vi "Generate_WayPoints_STOPMEASURE.vi"(8 "Update Position Loop Wait Time (us)":u32=50000, 11 "Input Cluster":T2={"Scan Rate (um/s)"=15.0, "X Start"=15.0, "X End"=15.0, "Y Start"=15.0, "Y End"=15.0, " Z Start"=15.0, "Number of Lines"=15, "V"=15.0, "Z End"=15.0, "Approach Rate (um/s)"=15.0, "Squish Approach Rate (um/s)"=15.0, "V 2"=15.0, "StopMeasureDist (um)"=15.0, "HoldTimer / us"=0}) -> (0 "output cluster":T1)   [LabVIEW 2023]
uses:
  TypeDefs/WayPointCluster.ctl
panel:
  in  "WayPointCluster":T1
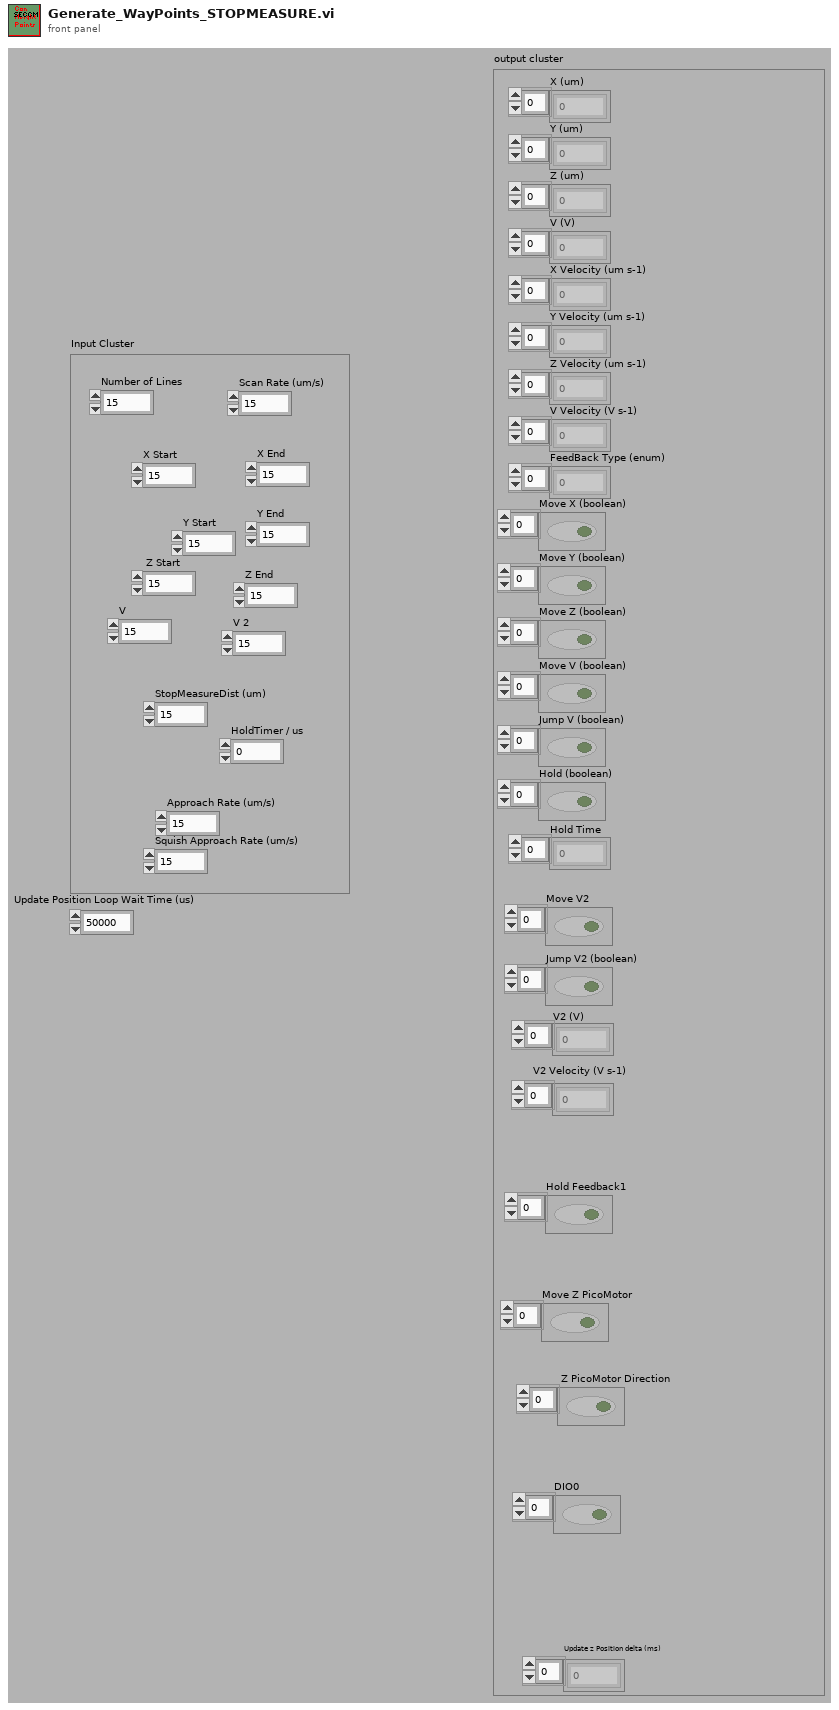
[diagram p1: front panel]
types:
  T1 = typedef "WayPointCluster.ctl" = cluster{"X (um)":dbl[], "Y (um)":dbl[], "Z (um)":dbl[], "V (V)":dbl[], "X Velocity (um s-1)":dbl[], "Y Velocity (um s-1)":dbl[], "Z Velocity (um s-1)":dbl[], "V Velocity (V s-1)":dbl[], "FeedBack Type (enum)":u16[], "Move X (boolean)":bool[], "Move Y (boolean)":bool[], "Move Z (boolean)":bool[], "Move V (boolean)":bool[], "Jump V (boolean)":bool[], "Hold (boolean)":bool[], "Hold Time":u32[], "V2 (V)":dbl[], "Move V2":bool[], "V2 Velocity (V s-1)":dbl[], "Jump V2 (boolean)":bool[], "Update z Position delta (ms)":i16[], "Hold Feedback1":bool[], "Move Z PicoMotor":bool[], " Z PicoMotor Direction":bool[], "DIO0":bool[]}
  T2 = cluster{"Scan Rate (um/s)":dbl, "X Start":dbl, "X End":dbl, "Y Start":dbl, "Y End":dbl, " Z Start":dbl, "Number of Lines":u32, "V":dbl, "Z End":dbl, "Approach Rate (um/s)":dbl, "Squish Approach Rate (um/s)":dbl, "V 2":dbl, "StopMeasureDist (um)":dbl, "HoldTimer / us":u32}
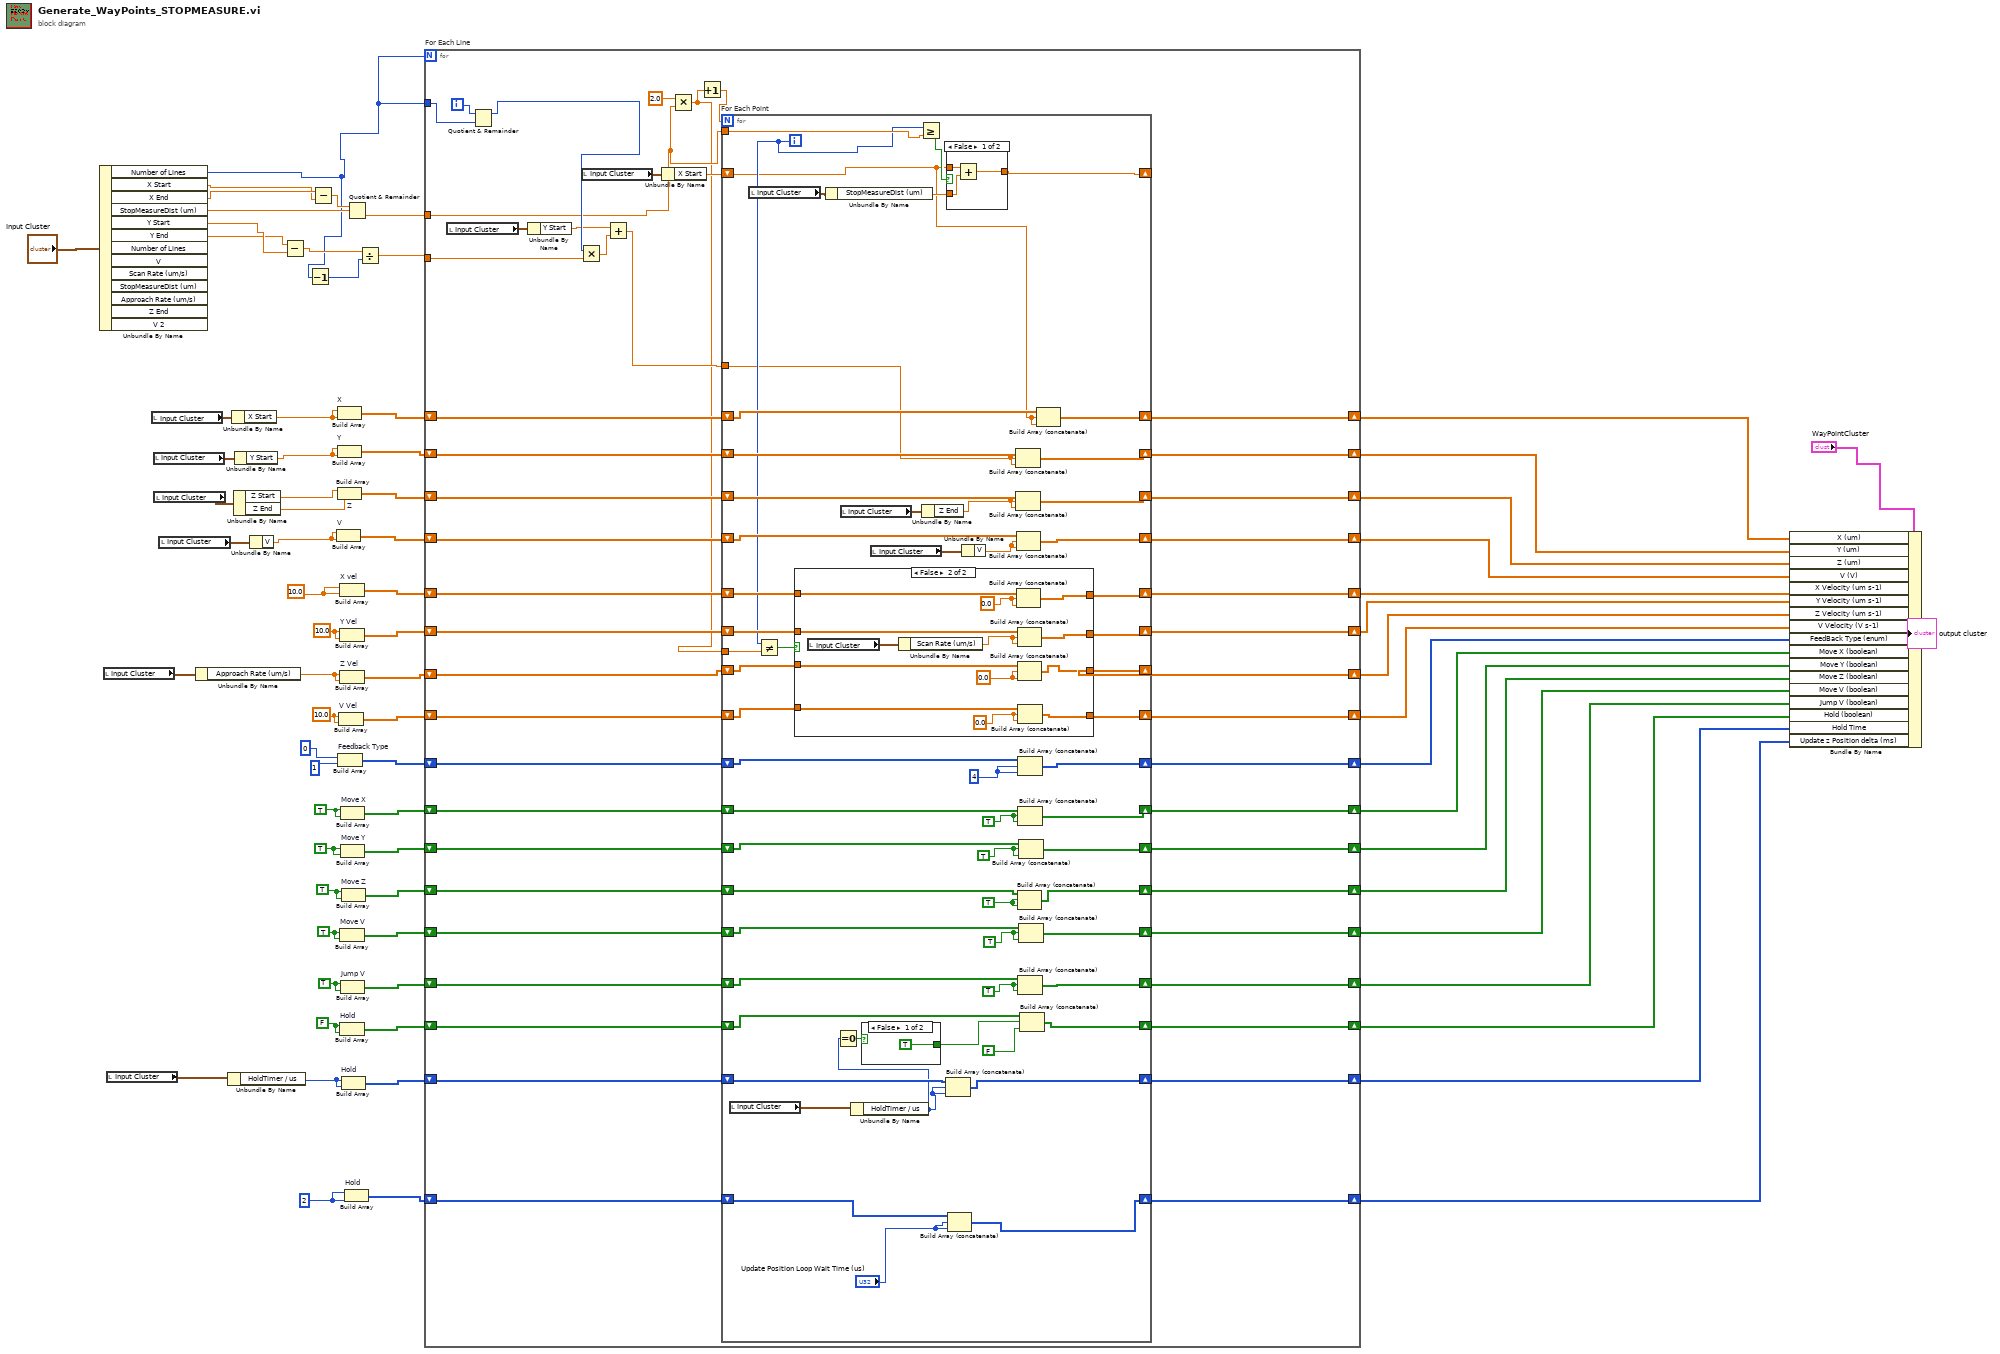
[diagram p0: block diagram]
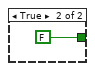
[diagram p2: hidden frame]
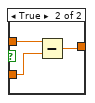
[diagram p3: hidden frame]
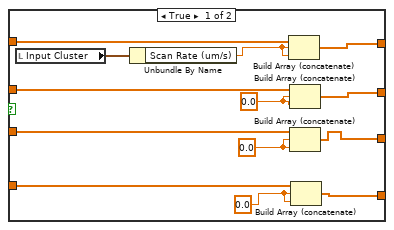
[diagram p4: hidden frame]
diagram:
  w3 = u32 2 ("element")
  w8 = FALSE
  w9 = TRUE
  w10 = TRUE
  w11 = TRUE
  w12 = TRUE
  w13 = TRUE
  w15 = 10.0 ("element")
  w17 = 10.0 ("element")
  w18 = 10.0 ("element")
  n1 = Unbundle By Name("Input Cluster") -> ("Number of Lines"=w64:u32, "X Start"=w62:dbl, "X End"=w72:dbl, "StopMeasureDist (um)"=w70:dbl, "Y Start"=w68:dbl, "Y End"=w67:dbl)  [unwired: 7 out]
  n2 = local read "Input Cluster"() -> (w41:T2)
  n3 = local read "Input Cluster"() -> (w35:T2)
  n4 = local read "Input Cluster"() -> (w45:T2)
  n5 = local read "Input Cluster"() -> (w44:T2)
  n6 = local read "Input Cluster"() -> (w43:T2)
  n7 = local read "Input Cluster"() -> (w42:T2)
  n8 = Unbundle By Name(w41) -> ("Approach Rate (um/s)"=w16:dbl)
  n9 = Unbundle By Name(w35) -> ("HoldTimer / us"=w7:u32)
  n10 = Unbundle By Name(w45) -> ("X Start"=w22:dbl)
  n11 = Unbundle By Name(w43) -> ("Z Start"=w20:dbl, "Z End"=w6:dbl)
  n12 = Unbundle By Name(w44) -> ("Y Start"=w21:dbl)
  n13 = Unbundle By Name(w42) -> ("V"=w19:dbl)
  n14 = Subtract(x=w67, y=w68) -> (x-y=w66:dbl)
  n15 = Decrement(x=w64) -> (x-1=w63:u32)
  n16 = Subtract(x=w72, y=w62) -> (x-y=w71:dbl)
  n17 = Build Array "V"(w19, w19) -> (w57:dbl[])
  n18 = Build Array "X"(w22, w22) -> (w60:dbl[])
  n19 = Build Array "Y"(w21, w21) -> (w59:dbl[])
  n20 = Build Array "Z"(w20, w6) -> (w58:dbl[])
  n21 = Build Array "Feedback Type"(u16 0 ("element"), u16 1 ("element")) -> (w52:u16[])
  n22 = Build Array "V Vel"(w15, w15) -> (w53:dbl[])
  n23 = Build Array "X vel"(w18, w18) -> (w56:dbl[])
  n24 = Build Array "Y Vel"(w17, w17) -> (w55:dbl[])
  n25 = Build Array "Z Vel"(w16, w16) -> (w54:dbl[])
  n26 = Build Array "Move V"(w10, w10) -> (w48:bool[])
  n27 = Build Array "Hold"(w8, w8) -> (w46:bool[])
  n28 = Build Array "Move X"(w13, w13) -> (w51:bool[])
  n29 = Build Array "Move Y"(w12, w12) -> (w50:bool[])
  n30 = Build Array "Jump V"(w9, w9) -> (w47:bool[])
  n31 = Build Array "Move Z"(w11, w11) -> (w49:bool[])
  n32 = Build Array "Hold"(w7, w7) -> (w36:u32[])
  n33 = Build Array "Hold"(w3, w3) -> (w2:u32[])
  n34 = Quotient & Remainder(x=w71, y=w70) -> (floor(x/y)=w69:dbl)  [unwired: 1 out]
  n35 = Divide(x=w66, y=w63) -> (x/y=w65:dbl)
  n36 = for "For Each Line" {
    N: w64 -> [_]
    tunnel: w69 -> [w79]
    tunnel: w64 -> [w120]
    tunnel: w65 -> [w119]
    shift-right: [w112] -> w40
    shift-left: w60 -> [w113]
    shift-right: [w97] -> w39
    shift-left: w59 -> [w111]
    shift-right: [w96] -> w38
    shift-left: w58 -> [w110]
    shift-right: [w95] -> w37
    shift-left: w57 -> [w109]
    shift-right: [w94] -> w34
    shift-left: w56 -> [w108]
    shift-right: [w93] -> w33
    shift-left: w55 -> [w107]
    shift-right: [w92] -> w32
    shift-left: w54 -> [w106]
    shift-right: [w91] -> w31
    shift-left: w53 -> [w105]
    shift-right: [w90] -> w30
    shift-left: w52 -> [w104]
    shift-right: [w89] -> w29
    shift-left: w51 -> [w103]
    shift-right: [w88] -> w28
    shift-left: w50 -> [w102]
    shift-right: [w87] -> w27
    shift-left: w49 -> [w101]
    shift-right: [w86] -> w26
    shift-left: w48 -> [w100]
    shift-right: [w85] -> w25
    shift-left: w47 -> [w99]
    shift-right: [w84] -> w24
    shift-left: w46 -> [w98]
    shift-right: [w76] -> w23
    shift-left: w36 -> [w77]
    shift-right: [w74] -> w1
    shift-left: w2 -> [w75]
    i -> [w121]
    n37 = local read "Input Cluster"() -> (w116:T2)
    n38 = Quotient & Remainder(x=w121, y=w120) -> (x-y*floor(x/y)=w118:u32)  [unwired: 1 out]
    n39 = Unbundle By Name(w116) -> ("Y Start"=w115:dbl)
    n40 = Multiply(x=w118, y=w119) -> (x*y=w117:dbl)
    n41 = local read "Input Cluster"() -> (w82:T2)
    n42 = Add(x=w115, y=w117) -> (x+y=w114:dbl)
    n43 = Unbundle By Name(w82) -> ("X Start"=w81:dbl)
    n44 = Multiply(x=2.0, y=w79) -> (x*y=w78:dbl)
    n45 = Increment(x=w78) -> (x+1=w80:dbl)
    n46 = for "For Each Point" {
      N: w80 -> [_]
      tunnel: w114 -> [w140]
      shift-right: [w179] -> w112
      shift-left: w113 -> [w180]
      shift-right: [w177] -> w97
      shift-left: w111 -> [w178]
      shift-right: [w175] -> w96
      shift-left: w110 -> [w176]
      shift-right: [w173] -> w95
      shift-left: w109 -> [w174]
      shift-right: [w171] -> w94
      shift-left: w108 -> [w172]
      shift-right: [w169] -> w93
      shift-left: w107 -> [w170]
      shift-right: [w167] -> w92
      shift-left: w106 -> [w168]
      shift-right: [w166] -> w91
      shift-left: w105 -> [w158]
      shift-right: [w165] -> w90
      shift-left: w104 -> [w157]
      shift-right: [w164] -> w89
      shift-left: w103 -> [w156]
      shift-right: [w163] -> w88
      shift-left: w102 -> [w155]
      shift-right: [w162] -> w87
      shift-left: w101 -> [w154]
      shift-right: [w161] -> w86
      shift-left: w100 -> [w153]
      shift-right: [w160] -> w85
      shift-left: w99 -> [w152]
      shift-right: [w159] -> w84
      shift-left: w98 -> [w151]
      tunnel: w78 -> [w147]
      shift-right: [w145] -> _
      shift-left: w81 -> [w141]
      tunnel: w79 -> [w144]
      shift-right: [w129] -> w76
      shift-left: w77 -> [w130]
      shift-right: [w125] -> w74
      shift-left: w75 -> [w127]
      i -> [w142]
      w132 = TRUE
      w133 = TRUE
      w134 = TRUE
      w135 = TRUE
      w136 = TRUE
      w137 = u16 4 ("element")
      n47 = local read "Input Cluster"() -> (w128:T2)
      n48 = local read "Input Cluster"() -> (w181:T2)
      n49 = Not Equal?(x=w142, y=w147) -> (x != y?=w148:bool)
      n50 = case shown="False" w148 {
        tunnel: w172 -> [w202 w215]
        tunnel: [w201 w214] -> w171
        tunnel: w170 -> [w200 w213]
        tunnel: [w199 w212] -> w169
        tunnel: w168 -> [w198 w211]
        tunnel: [w197 w210] -> w167
        tunnel: [w196 w209] -> w166
        tunnel: w158 -> [w195 w208]
        frame True {
          w190 = 0.0 ("element")
          w191 = 0.0 ("element")
          w192 = 0.0 ("element")
          n51 = local read "Input Cluster"() -> (w194:T2)
          n52 = Unbundle By Name(w194) -> ("Scan Rate (um/s)"=w193:dbl)
          n53 = Build Array (concatenate) ("X")(w202, w193, w193) -> (w201:dbl[])
          n54 = Build Array (concatenate) ("X")(w200, w192, w192) -> (w199:dbl[])
          n55 = Build Array (concatenate) ("X")(w198, w191, w191) -> (w197:dbl[])
          n56 = Build Array (concatenate) ("X")(w195, w190, w190) -> (w196:dbl[])
        }
        frame False {
          w203 = 0.0 ("element")
          w204 = 0.0 ("element")
          w206 = 0.0 ("element")
          n57 = local read "Input Cluster"() -> (w207:T2)
          n58 = Unbundle By Name(w207) -> ("Scan Rate (um/s)"=w205:dbl)
          n59 = Build Array (concatenate) ("X")(w215, w206, w206) -> (w214:dbl[])
          n60 = Build Array (concatenate) ("X")(w213, w205, w205) -> (w212:dbl[])
          n61 = Build Array (concatenate) ("X")(w211, w204, w204) -> (w210:dbl[])
          n62 = Build Array (concatenate) ("X")(w208, w203, w203) -> (w209:dbl[])
        }
      }
      n63 = Unbundle By Name(w181) -> ("StopMeasureDist (um)"=w146:dbl)
      n64 = local read "Input Cluster"() -> (w150:T2)
      n65 = Unbundle By Name(w128) -> ("HoldTimer / us"=w122:u32)
      n66 = Equal To 0?(x=w122) -> (x = 0?=w123:bool)
      n67 = case shown="False" w123 {
        tunnel: [TRUE FALSE] -> w124
        frame False {
        }
        frame True {
        }
      }
      n68 = local read "Input Cluster"() -> (w149:T2)
      n69 = Greater Or Equal?(x=w142, y=w144) -> (x >= y?=w143:bool)
      n70 = Unbundle By Name(w150) -> ("Z End"=w139:dbl)
      n71 = Build Array (concatenate) ("X")(w130, w122, w122) -> (w129:u32[])
      n72 = case shown="False" w143 {
        tunnel: w146 -> [w186 w189]
        tunnel: w141 -> [w185 w187]
        tunnel: [w184 w188] -> w145
        frame False {
          n73 = Add(x=w185, y=w186) -> (x+y=w184:dbl)
        }
        frame True {
          n74 = Subtract(x=w187, y=w189) -> (x-y=w188:dbl)
        }
      }
      n75 = Build Array (concatenate) ("X")(w127, "Update Position Loop Wait Time (us)", "Update Position Loop Wait Time (us)") -> (w125:u32[])
      n76 = Unbundle By Name(w149) -> ("V"=w138:dbl)
      n77 = Build Array (concatenate) ("X")(w178, w140, w140) -> (w177:dbl[])
      n78 = Build Array (concatenate) ("X")(w176, w139, w139) -> (w175:dbl[])
      n79 = Build Array (concatenate) ("X")(w174, w138, w138) -> (w173:dbl[])
      n80 = Build Array (concatenate) ("X")(w154, w134, w134) -> (w162:bool[])
      n81 = Build Array (concatenate) ("X")(w157, w137, w137) -> (w165:u16[])
      n82 = Build Array (concatenate) ("X")(w156, w136, w136) -> (w164:bool[])
      n83 = Build Array (concatenate) ("X")(w152, w132, w132) -> (w160:bool[])
      n84 = Build Array (concatenate) ("X")(w155, w135, w135) -> (w163:bool[])
      n85 = Build Array (concatenate) ("X")(w153, w133, w133) -> (w161:bool[])
      n86 = Build Array (concatenate) ("X")(w151, w124, FALSE) -> (w159:bool[])
      n87 = Build Array (concatenate) ("X")(w180, w141, w141) -> (w179:dbl[])
    }
  }
  n88 = Bundle By Name(cluster="WayPointCluster", "X (um)"=w40, "Y (um)"=w39, "Z (um)"=w38, "V (V)"=w37, "X Velocity (um s-1)"=w34, "Y Velocity (um s-1)"=w33, "Z Velocity (um s-1)"=w32, "V Velocity (V s-1)"=w31, "FeedBack Type (enum)"=w30, "Move X (boolean)"=w29, "Move Y (boolean)"=w28, "Move Z (boolean)"=w27, "Move V (boolean)"=w26, "Jump V (boolean)"=w25, "Hold (boolean)"=w24, "Hold Time"=w23, "Update z Position delta (ms)"=w1) -> (→"output cluster":T1)
